vi "Configure.vi"(8 "error in":errorcluster, 10 "ConfigRef In":T1, 11 "TC01 in":refnum<class "TC01.lvclass">) -> (0 "error out":errorcluster, 3 "TC01 out":refnum<class "TC01.lvclass">)   [LabVIEW 2015, in "TC01.lvclass"]
uses:
  TC01.lvclass
  <vilib>/Utility/config.llb/Config Data RefNum.ctl
  TC01.lvclass/TC01.ctl
  <vilib>/Utility/config.llb/Read Key (String).vi
  <vilib>/Utility/config.llb/Read Key (Double).vi
  <vilib>/Utility/config.llb/Read Key (I32).vi
  <vilib>/DAQmx/create/channels.llb/DAQmx Create Channel (AI-Temperature-Thermocouple).vi
  <vilib>/Utility/config.llb/NI_LVConfig.lvlib
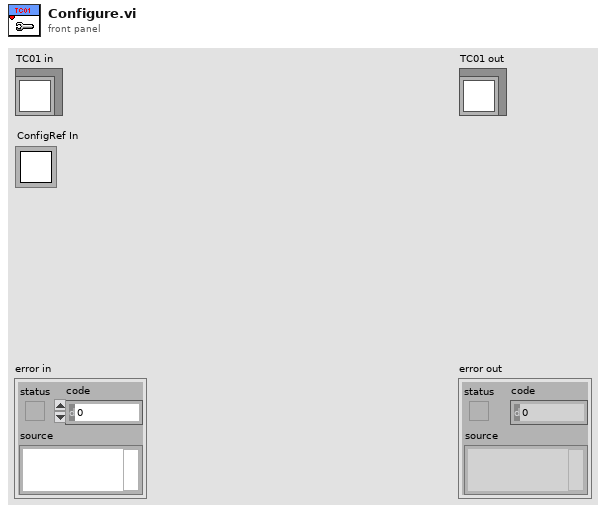
[diagram p1: front panel]
types:
  T1 = typedef "NI_LVConfig.lvlib/Config Data RefNum.ctl" = refnum<k1>
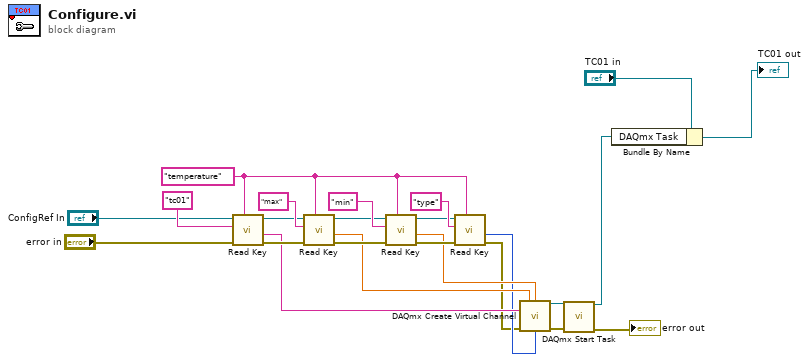
[diagram p0: block diagram]
diagram:
  w23 = "temperature" ("section")
  n1 = call-poly <vilib>:"Read Key.vi"("section"=w23, "error in (no error)"="error in", "key"="tc01", "refnum"="ConfigRef In") -> ("error out"=w16:errorcluster, "value"=w14:string, "refnum out"=w15:T1)  [unwired: 4 in, 1 out]
  n2 = call-poly <vilib>:"Read Key.vi"("section"=w23, "error in (no error)"=w16, "key"="max", "refnum"=w15) -> ("error out"=w19:errorcluster, "value"=w12:dbl, "refnum out"=w18:T1)  [unwired: 4 in, 1 out]
  n3 = call-poly <vilib>:"Read Key.vi"("section"=w23, "error in (no error)"=w19, "key"="min", "refnum"=w18) -> ("error out"=w22:errorcluster, "value"=w11:dbl, "refnum out"=w21:T1)  [unwired: 4 in, 1 out]
  n4 = call-poly <vilib>:"Read Key.vi"("section"=w23, "error in (no error)"=w22, "key"="type", "refnum"=w21) -> ("error out"=w7:errorcluster, "value"=w10:i32)  [unwired: 4 in, 2 out]
  n5 = call-poly <vilib>:"DAQmx Create Virtual Channel.vi"("maximum value"=w12, "minimum value"=w11, "physical channels"=w14, "error in"=w7, "thermocouple type"=w10) -> ("task out"=w9:refnum<k21>, "error out"=w8:errorcluster)  [unwired: 9 in]
  n6 = call <vilib>:"DAQmx Start Task.vi"("task/channels in"=w9, "error in"=w8) -> ("task out"=w4:refnum<k21>, "error out"=→"error out":errorcluster)  [unwired: 12 in]
  n7 = Bundle By Name(cluster="TC01 in", "DAQmx Task"=w4) -> (→"TC01 out":refnum<class "TC01.lvclass">)
